vi "Find Default Events Path.vi"(8 "error in":errorcluster, 10 "Event":string, 11 "DQMH Library Ref":refnum<vi>) -> (0 "error out":errorcluster, 3 "Event Path":path)   [LabVIEW 2019, in "Panther Dashboard.lvlib"]
uses:
  Panther Dashboard.lvlib
  <vilib>/Utility/error.llb/Error Cluster From Error Code.vi
  <vilib>/ErrorRing/Error Ring.xnode
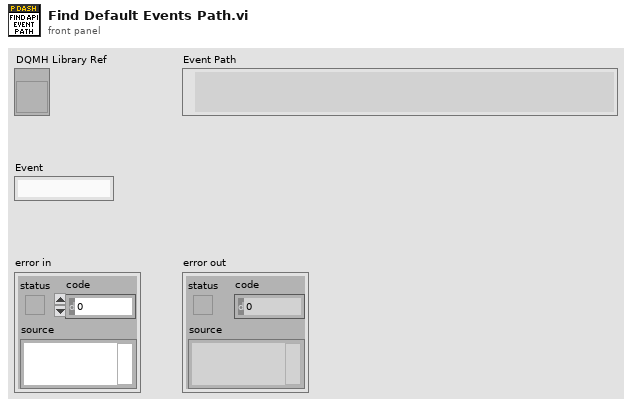
[diagram p1: front panel]
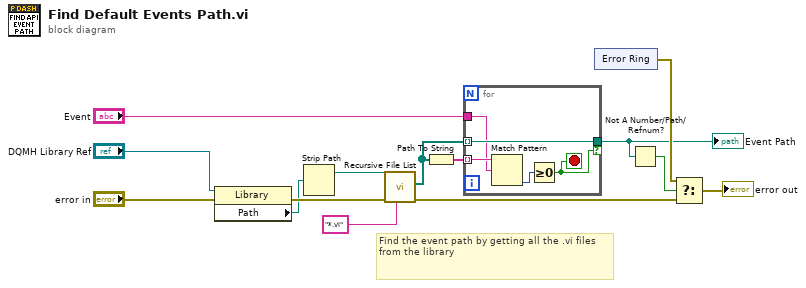
[diagram p0: block diagram]
diagram:
  # "Find the event path by getting all the .vi files\nfrom the library"
  n1 = property class="Library"(reference="DQMH Library Ref", error in="error in") -> (error out=w10:errorcluster, "Path"=w3:path)  [unwired: 1 out]
  n2 = Strip Path(path=w3) -> (stripped path=w4:path)  [unwired: 1 out]
  n3 = call <vilib>:"Recursive File List.vi"("pattern"="*.vi", "error in (no error)"=w10, "Folder Path"=w4) -> ("error out"=w11:errorcluster, "All Files in Dir"=w5:path[])  [unwired: 4 in, 3 out]
  n4 = Path To String(path=w5) -> (string=w1:string[])
  n5 = for {
    tunnel: w1 -> [w18] mode=indexing
    tunnel: w5 -> [w19] mode=indexing
    tunnel: [w19] -> w9 if=w16
    tunnel: "Event" -> [w15]
    stop <- w16 stop-if-true
    n6 = Match Pattern(string=w18, regular expression=w15) -> (offset past match=w17:i32)  [unwired: 1 in, 3 out]
    n7 = Greater Or Equal To 0?(x=w17) -> (x >= 0?=w16:bool)
  }
  "Event Path" <- w9
  n8 = xnode "Error Ring"() -> ("error out"=w12:errorcluster)
  n9 = Not A Number/Path/Refnum?(number/path/refnum=w9) -> (NaN/Path/Refnum?=w2:bool)
  n10 = Select(t=w12, s=w2, f=w11) -> (s? t:f=→"error out":errorcluster)
